vi "PH_ImageCoG_Plotter.get Cam instances.vi"(0 "i ref in":refnum<vi>, 5 "error in":errorcluster) -> (14 "i ref out":refnum<vi>, 19 "error out":errorcluster)   [LabVIEW 2014, in "PH_ImageCoG_Plotter.lvlib"]
doc: "This VI gets the camaras instanciated locally and writes them to own attributes and the GUI element."
uses:
  PH_ImageCoG_Plotter.lvlib
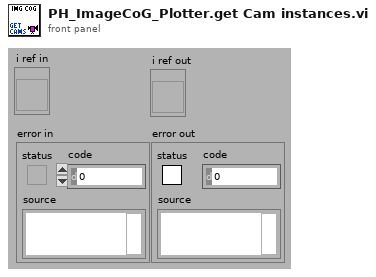
[diagram p1: front panel]
types:
  T1 = typedef "PH_ImageCoG_Plotter.lvlib/PH_ImageCoG_Plotter.i attribute.ctl" = cluster{"GUI Refs":cluster{"Delete":refnum<vi>, "Calibration status":refnum<vi>, "BI subtracted":refnum<vi>, "calc Beam Anal":refnum<vi>, "CoG - x":refnum<vi>, "CoG - y":refnum<vi>, "Type":refnum<vi>, "Center":refnum<vi>, "exp - X":refnum<vi>, "exp - Y":refnum<vi>, "Delta - X":refnum<vi>, "Delta - Y":refnum<vi>, "Available Cams":refnum<vi>, "CoG X":refnum<vi>, "CoG Y":refnum<vi>, "Delta X":refnum<vi>, "Delta Y":refnum<vi>, "Export Data":refnum<vi>, "Calibration data":refnum<vi>}, "Calibration":cluster{"Status":T2, "Calibration data":T3, "Calibration Data File":path}, "Beam Analysis":cluster{"on":bool, "exp - X":i32, "exp - Y":i32, "Type":bool, "Data":cluster{"current time":timestamp, "CoG-x":dbl, "CoG-y":dbl, "Delta-x":dbl, "Delta-y":dbl}[], "Datasets strored":i32, "Dataarray Size":i32}, "Cam instances":string[], "DIM Service Events":T4[], "Images":cluster{"Background":T7, "OP":T7, "GUI":T7}}
  T2 = typedef "PH_StatusHandler.lvlib/PH_StatusHandler.Status.ctl" = i16
  T3 = typedef "PH_ImageCalibrator.lvlib/PH_ImageCalibrator.Calibration Data.ctl" = cluster{"Date":string, "Time":string, "Cam Settings":cluster{"Cam ID":string, "Gain":dbl, "Brightness":dbl, "Shutter":dbl, "Cam Error":bool, "Mode":i32}, "Background Image":cluster{"Image":dbl[][], "Image Error":bool}, "Linear Calibration":cluster{"Calibration Factor":dbl, "not mm or mrad":bool}, "Energy Calibration":cluster{"Calibration Factor":dbl, "no mJ":bool}}
  T4 = typedef "BaseProcess.lvlib/BaseProcess.event definition.ctl" = cluster{"CAEEvtDef":T5, "Data Descriptor":T6}
  T5 = typedef "CAEObj.lvlib/CAEObj.event definition.ctl" = cluster{"URL":string, "enable":bool, "ignoreResID":bool}
  T6 = typedef "BaseProcess.lvlib/BaseProcess.descriptor string definition.ctl" = string
  T7 = typedef "IMAQ Image.ctl" = refnum<image>
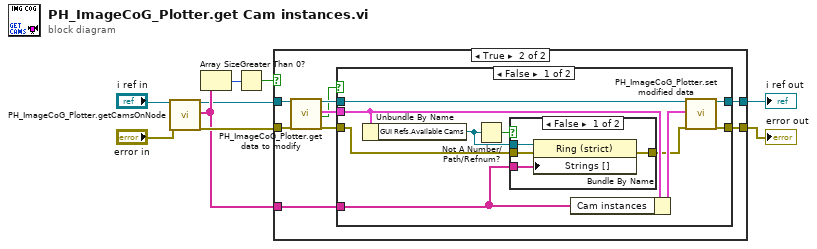
[diagram p0: block diagram]
diagram:
  n1 = call "PH_ImageCoG_Plotter.getCamsOnNode.vi"("i ref in"="i ref in", "error in (no error)"="error in") -> ("i ref out"=w1:refnum<vi>, "cams on node"=w3:string[], "error out"=w7:errorcluster)  [unwired: 15 in]
  n2 = Array Size(array=w3) -> (size(s)=w6:i32)
  n3 = Greater Than 0?(x=w6) -> (x > 0?=w5:bool)
  n4 = case shown="True" w5 {
    tunnel: w7 -> [w11 w15]
    tunnel: [w11 w14] -> w9
    tunnel: w1 -> [w10 w13]
    tunnel: [w10 w16] -> w8
    tunnel: w3 -> [_ w12]
    frame False {
    }
    frame True {
      n5 = call "PH_ImageCoG_Plotter.get data to modify.vi"("i ref in"=w13, "error in (no error)"=w15) -> ("i ref out"=w20:refnum<vi>, "i attribute"=w18:T1, "timed out"=w17:bool, "error out"=w19:errorcluster)  [unwired: 14 in]
      n6 = case shown="False" w17 {
        tunnel: w20 -> [w30 w37]
        tunnel: w19 -> [w24 w36]
        tunnel: [w29 w36] -> w14
        tunnel: [w28 w37] -> w16
        tunnel: w18 -> [w26 _]
        tunnel: w12 -> [w25 _]
        frame False {
          n7 = Unbundle By Name(w26) -> ("GUI Refs.Available Cams"=w21:refnum<vi>)
          n8 = Not A Number/Path/Refnum?(number/path/refnum=w21) -> (NaN/Path/Refnum?=w22:bool)
          n9 = case shown="False" w22 {
            tunnel: w21 -> [w34 _]
            tunnel: w25 -> [w33 _]
            tunnel: w24 -> [w32 w35]
            tunnel: [w31 w35] -> w23
            frame False {
              n10 = property class="Ring (strict)"(reference=w34, error in=w32, "Strings []"=w33) -> (error out=w31:errorcluster)  [unwired: 1 out]
            }
            frame True {
            }
          }
          n11 = Bundle By Name(cluster=w26, "Cam instances"=w25) -> (w27:T1)
          n12 = call "PH_ImageCoG_Plotter.set modified data.vi"("i ref in"=w30, "i attribute"=w27, "error in (no error)"=w23) -> ("i ref out"=w28:refnum<vi>, "error out"=w29:errorcluster)  [unwired: 15 in]
        }
        frame True {
        }
      }
    }
  }
  "i ref out" <- w8
  "error out" <- w9
